vi "KG set cw sp.vi"(8 "Fehler (Eingang, kein Fehler)":errorcluster, 9 "Concentration":dbl, 10 "pump":u32, 11 "VISA-Ressourcenname":refnum<visa-resource-name>) -> (0 "Fehler (Ausgang)":errorcluster, 2 "Kommando gesendet":string, 3 "VISA-Ressourcenname (Ausgang)":refnum<visa-resource-name>)   [LabVIEW 2020, in "Linearisierung v2.lvlib" / "Gasteiler.lvlib" / "HovaCAL_Interface.lvlib" / "KGN.lvlib" / "set.lvlib"]
uses:
  set.lvlib
  KGN.lvlib
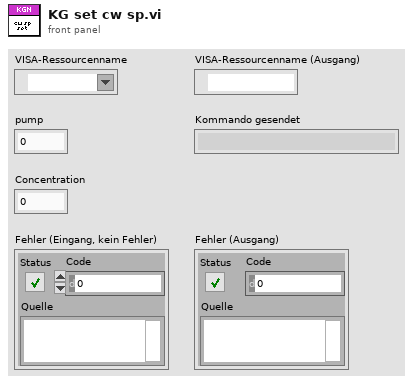
[diagram p1: front panel]
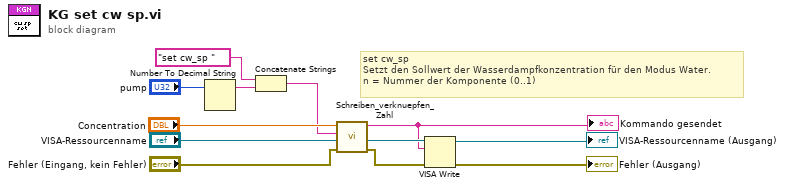
[diagram p0: block diagram]
diagram:
  # "set cw_sp\nSetzt den Sollwert der Wasserdampfkonzentration für den Modus Water.\nn = Nummer der Komponente (0..1)"
  n1 = Number To Decimal String(number="pump") -> (decimal integer string=w6:string)  [unwired: 1 in]
  n2 = Concatenate Strings("set cw_sp " ("Schreibpuffer"), w6) -> (w1:string)
  n3 = call "Schreiben_verknuepfen_Zahl.vi"("error in (no error)"="Fehler (Eingang, kein Fehler)", "Order"=w1, "Zahl"="Concentration") -> ("error out"=w4:errorcluster, "Verknüpfter String"=w3:string)  [unwired: 7 in]
  "Kommando gesendet" <- w3
  n4 = VISA Write(VISA resource name="VISA-Ressourcenname", write buffer=w3, error in (no error)=w4) -> (VISA resource name out=→"VISA-Ressourcenname (Ausgang)":refnum<visa-resource-name>, error out=→"Fehler (Ausgang)":errorcluster)  [unwired: 1 out]
